vi "UART Write.vi"   [LabVIEW 2020, in "LMH-LINX.lvlib"]
uses:
  LMH-LINX.lvlib
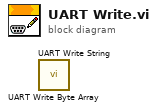
[diagram p0: block diagram]
diagram:
  n1 = call "UART Write Byte Array.vi"() -> ()  [unwired: 10 in, 2 out]
  n2 = call "UART Write String.vi"() -> ()  [unwired: 10 in, 2 out]
